vi "XIPIN_Memory_Interface_Generator_(MIG_7_Series)_2_4.vi"   [LabVIEW 2017]
doc: "This Memory Interface Generator is a simple menu driven tool to generate advanced memory interfaces. This tool generates HDL and pin placement constraints that will help you design your application. Kintex-7 supports DDR3 SDRAM, DDR2 SDRAM, LPDDR2 SDRAM, QDR II+ SRAM, RLDRAMII and RLDRAMIII. Virtex-7 supports DDR3 SDRAM, DDR2 SDRAM, LPDDR2 SDRAM, QDR II+ SRAM, RLDRAMII and RLDRAMIII. Artix-7 supports DDR3 SDRAM, DDR2 SDRAM and LPDDR2 SDRAM. Zynq supports DDR3 SDRAM, DDR2 SDRAM and LPDDR2 SDRAM\n------------------------------------\n<b>Need License</b> : No\n<b>Interface</b> : AXI4"
uses:
  <vilib>/rvi/XilinxIP/XIPIN_XNode/niFpgaXIPIN.xnode
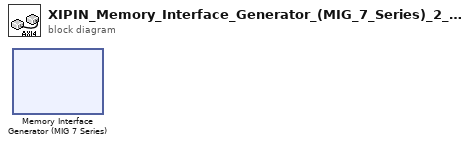
[diagram p0: block diagram]
diagram:
  n1 = xnode ("Memory Interface Generator (MIG 7 Series)")() -> ()
